vi "midi_CloseInstruments.vi"(8 "error in (no error)":errorcluster, 11 "vi references":refnum<vi>[](array[refnum])) -> (0 "error out":errorcluster)   [LabVIEW 2013]
doc: "Close the subVIs (instruments) of the band."
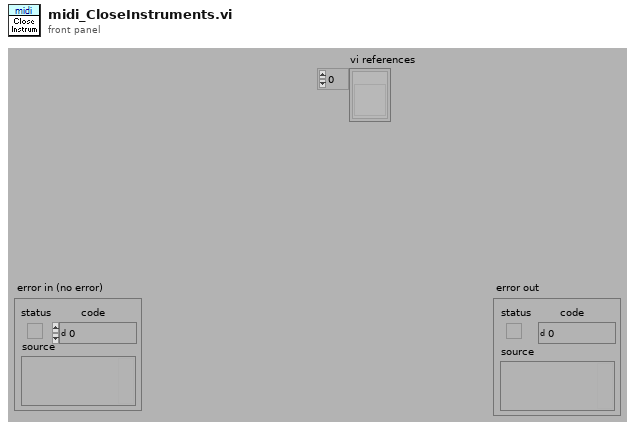
[diagram p1: front panel]
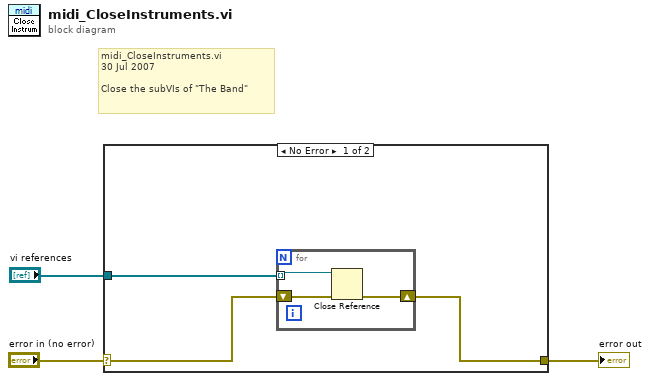
[diagram p0: block diagram]
diagram:
  # "midi_CloseInstruments.vi\n30 Jul 2007\n\nClose the subVIs of \"The Band\""
  n1 = case shown="No Error" "error in (no error)" {
    selector: "error in (no error)" -> [w5 w10]
    tunnel: [w4 w10] -> w2
    tunnel: "vi references" -> [w6 _]
    frame No Error {
      n2 = for {
        tunnel: w6 -> [w9] mode=indexing
        shift-right: [w7] -> w4
        shift-left: w5 -> [w8]
        n3 = Close Reference(reference=w9, error in (no error)=w8) -> (error out=w7:errorcluster)
      }
    }
    frame Error {
    }
  }
  "error out" <- w2
